vi "Toggle Menu State.vi"(8 "error in (no error)":errorcluster, 11 "MenuButton in":refnum<class "MenuButton.lvclass">) -> (0 "error out":errorcluster, 2 "Menu Bottom Position":u32, 3 "MenuButton out":refnum<class "MenuButton.lvclass">)   [LabVIEW 2017, in "MenuButtons.lvlib" / "MenuButton.lvclass"]
uses:
  MenuButton.lvclass
  MenuButton.lvclass/MenuButton.ctl
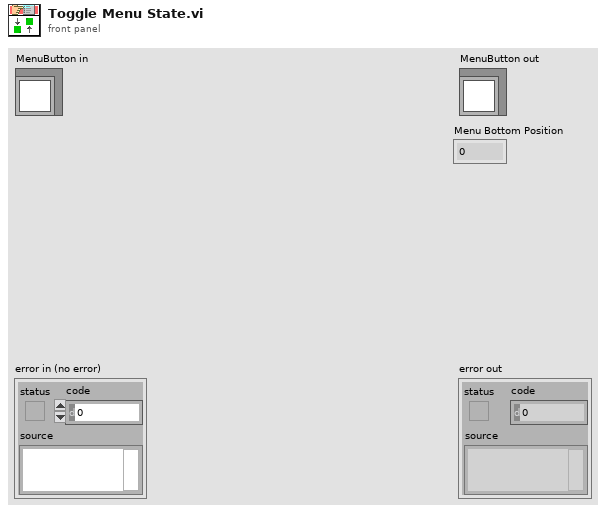
[diagram p1: front panel]
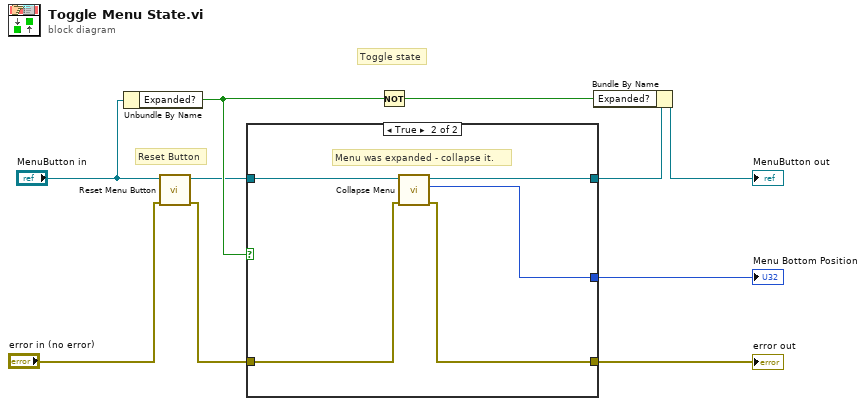
[diagram p0: block diagram]
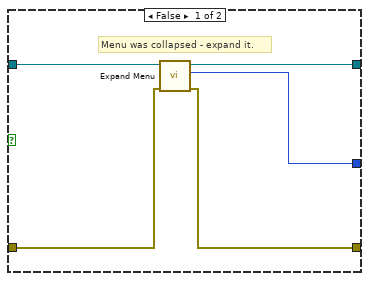
[diagram p2: hidden frame]
diagram:
  # "Toggle state"
  # "Reset Button"
  n1 = Unbundle By Name("MenuButton in") -> ("Expanded?"=w10:bool)
  n2 = call "Reset Menu Button.vi"("error in (no error)"="error in (no error)", "MenuButton in"="MenuButton in") -> ("error out"=w3:errorcluster, "MenuButton out"=w5:refnum<class "MenuButton.lvclass">)  [unwired: 8 in]
  n3 = case shown="True" w10 {
    tunnel: w5 -> [w15 w20]
    tunnel: [w14 w19] -> w9
    tunnel: w3 -> [w13 w18]
    tunnel: [w12 w17] -> w2
    tunnel: [w11 w16] -> w1
    frame False {
      # "Menu was collapsed - expand it."
      n4 = call "Expand Menu.vi"("error in (no error)"=w13, "MenuButton in"=w15) -> ("error out"=w12:errorcluster, "Ending Bottom Position"=w11:u32, "MenuButton out"=w14:refnum<class "MenuButton.lvclass">)  [unwired: 7 in]
    }
    frame True {
      # "Menu was expanded - collapse it."
      n5 = call "Collapse Menu.vi"("error in (no error)"=w18, "MenuButton in"=w20) -> ("error out"=w17:errorcluster, "Menu Bottom Position"=w16:u32, "MenuButton out"=w19:refnum<class "MenuButton.lvclass">)  [unwired: 7 in]
    }
  }
  "error out" <- w2
  "Menu Bottom Position" <- w1
  n6 = Not(x=w10) -> (.not. x?=w7:bool)
  n7 = Bundle By Name(cluster=w9, "Expanded?"=w7) -> (→"MenuButton out":refnum<class "MenuButton.lvclass">)
